vi "parse_RxMessage(SAP).vi"(11 "ReadBuffer In":u8[](array[numeric])) -> (0 "msg size":u32, 1 "ip src":u32, 2 "IrigTime":T1, 3 "Message Data":u8[](array[numeric]), 4 "udp src port":u32)   [LabVIEW 2020, in "AIM664LV.lvlib"]
uses:
  AIM664LV.lvlib
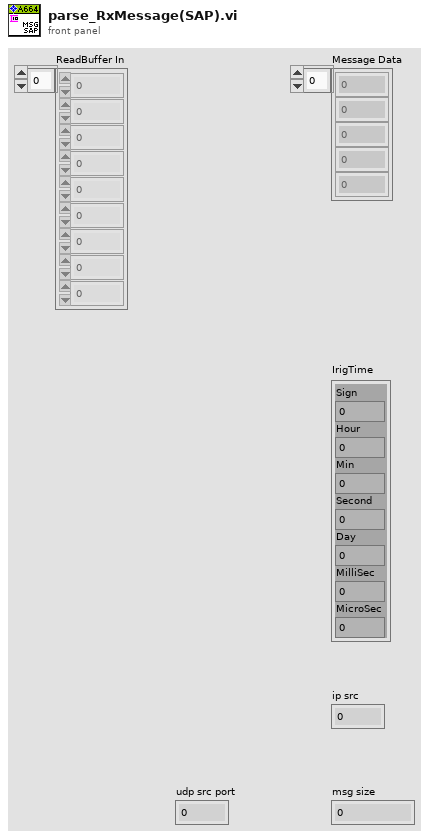
[diagram p1: front panel]
types:
  T1 = cluster{"Sign":i32, "Hour":u32, "Min":u32, "Second":u32, "Day":u32, "MilliSec":u32, "MicroSec":u32}
  T2 = typedef "AIM664LV.lvlib/IrigTime.ctl" = cluster{"Sign":i32, "Day":u32, "Hour":u32, "Min":u32, "Second":u32, "MilliSec":u32, "MicroSec":u32}
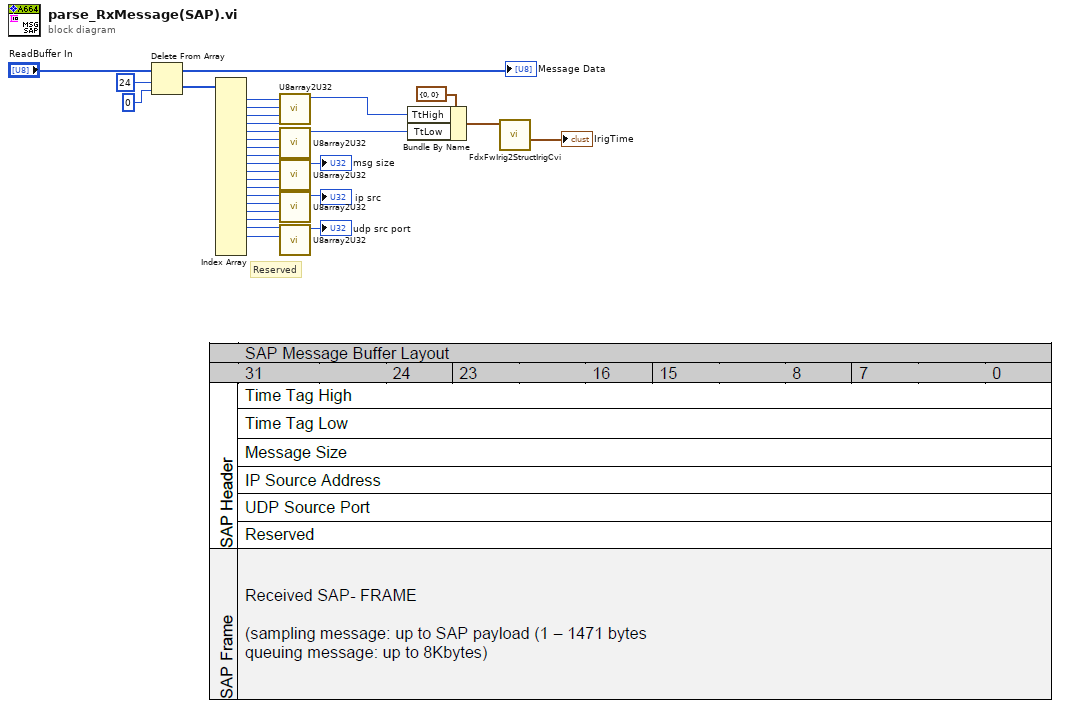
[diagram p0: block diagram]
diagram:
  # "Reserved"
  n1 = Delete From Array(array="ReadBuffer In", length=24, index=0) -> (deleted portion=w20:u8[], array with subset deleted=→"Message Data":u8[])
  n2 = Index Array(array=w20) -> (element #1=w24:u8, element #2=w23:u8, element #3=w22:u8, element #4=w21:u8, element #5=w17:u8, element #6=w16:u8, element #7=w15:u8, element #8=w14:u8, element #9=w13:u8, element #10=w12:u8, element #11=w11:u8, element #12=w10:u8, element #13=w9:u8, element #14=w8:u8, element #15=w7:u8, element #16=w6:u8, element #17=w3:u8, element #18=w2:u8)  [unwired: 20 in, 2 out]
  n3 = call "U8array2U32.vi"("hi 2"=w21, "lo 2"=w22, "hi"=w23, "lo"=w24) -> ("(hi.lo)"=w19:u32)  [unwired: 7 in]
  n4 = call "U8array2U32.vi"("hi 2"=w14, "lo 2"=w15, "hi"=w16, "lo"=w17) -> ("(hi.lo)"=w18:u32)  [unwired: 7 in]
  n5 = call "U8array2U32.vi"("hi 2"=w10, "lo 2"=w11, "hi"=w12, "lo"=w13) -> ("(hi.lo)"=→"msg size":u32)  [unwired: 7 in]
  n6 = call "U8array2U32.vi"("hi 2"=w6, "lo 2"=w7, "hi"=w8, "lo"=w9) -> ("(hi.lo)"=→"ip src":u32)  [unwired: 7 in]
  n7 = call "U8array2U32.vi"("hi"=w2, "lo"=w3) -> ("(hi.lo)"=→"udp src port":u32)  [unwired: 9 in]
  n8 = Bundle By Name(cluster=cluster{"TtHigh":u32, "TtLow":u32} {"TtHigh"=0, "TtLow"=0} ("FwIrigTime"), "TtHigh"=w19, "TtLow"=w18) -> (w26:cluster{"TtHigh":u32, "TtLow":u32})
  n9 = call "FdxFwIrig2StructIrigCvi.vi"("FwIrigTime"=w26) -> ("IrigTime"=→"IrigTime":T2)  [unwired: 9 in, 1 out]
